vi "Scan Setup.vi"(8 "error in (no error)":errorcluster, 11 "Function Gen Scan in":refnum<class "Function Gen Scan.lvclass">) -> (0 "error out":errorcluster, 3 "Function Gen Scan out":refnum<class "Function Gen Scan.lvclass">)   [LabVIEW 2017, in "Function Gen Scan.lvclass"]
doc: "Configure the instrument based on the class member data. This step comes after the user has closed the \"Scan Setup\" window and before the actual scan -- so instruments are configured with the user's specified settings."
uses:
  Function Gen Scan.lvclass
  Function Gen Scan.lvclass/Function Gen Scan.ctl
  Scanner/Scanner.lvclass
  Instruments/Utility Classes/Scannable/Scannable.lvclass
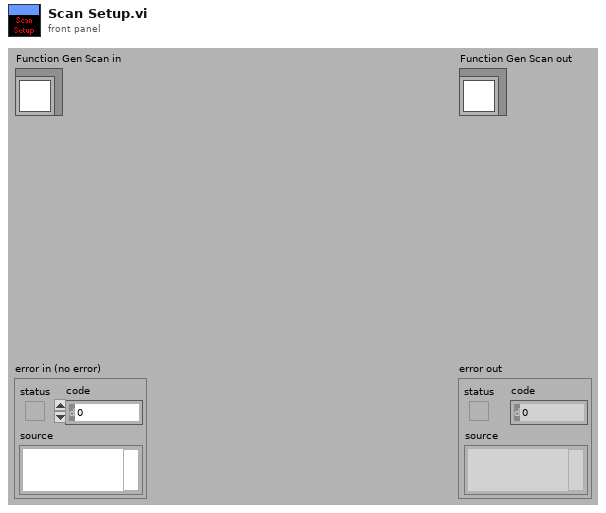
[diagram p1: front panel]
types:
  T1 = typedef "Channel.ctl" = u16
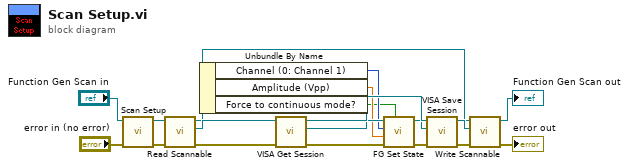
[diagram p0: block diagram]
diagram:
  n1 = call-parent "Scan Setup.vi"("error in (no error)"="error in (no error)", "Scanner in"="Function Gen Scan in") -> ("error out"=w9:errorcluster, "Scanner out"=w14:refnum<class "Function Gen Scan.lvclass">)  [unwired: 8 out]
  n2 = call-dynamic "Read Scannable.vi"("error in (no error)"=w9, "Scanner.lvclass in"=w14) -> ("error out"=w10:errorcluster, "Scannable.lvclass"=w17:refnum<class "Scannable.lvclass">, "Scanner.lvclass out"=w8:refnum<class "Function Gen Scan.lvclass">)  [unwired: 7 out]
  n3 = Unbundle By Name(w8) -> ("Channel (0: Channel 1)"=w6:T1, "Amplitude (Vpp)"=w5:dbl[unit], "Force to continuous mode?"=w3:bool)
  n4 = call-dynamic "VISA Get Session.vi"("error in (no error)"=w10, "Instrument.lvclass in"=w17) -> ("error out"=w4:errorcluster, "VISA Resource Name"=w7:refnum<visa-resource-name>, "Instrument.lvclass out"=w16:refnum<class "Scannable.lvclass">)  [unwired: 7 out]
  n5 = call "FG Set State.vi"("Force to continuous mode?"=w3, "error in (no error)"=w4, "voltage (Vpp)"=w5, "Channel (0: Channel 1)"=w6, "VISA resource name"=w7) -> ("error out"=w1:errorcluster, "VISA resource name out"=w2:refnum<visa-resource-name>)  [unwired: 5 in]
  n6 = call-dynamic "VISA Save Session.vi"("error in (no error)"=w1, "VISA Resource Name"=w2, "Instrument.lvclass in"=w16) -> ("error out"=w12:errorcluster, "Instrument.lvclass out"=w15:refnum<class "Scannable.lvclass">)  [unwired: 7 out]
  n7 = call-dynamic "Write Scannable.vi"("error in (no error)"=w12, "Scannable.lvclass"=w15, "Scanner.lvclass in"=w8) -> ("error out"=→"error out":errorcluster, "Scanner.lvclass out"=→"Function Gen Scan out":refnum<class "Function Gen Scan.lvclass">)  [unwired: 7 out]
